vi "GetDataTypeDescription.vi"(8 "error in (no error)":errorcluster, 11 "Variant":variant) -> (0 "error out":errorcluster, 3 "String":string)   [LabVIEW 2014]
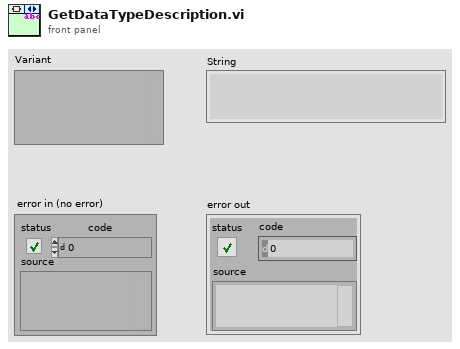
[diagram p1: front panel]
types:
  T1 = typedef "Type Descriptor__ogtk.ctl" = i16[]
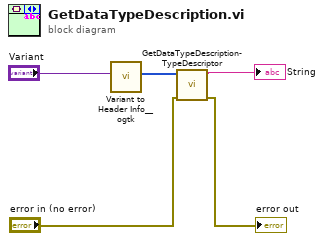
[diagram p0: block diagram]
diagram:
  n1 = call <userlib>:"Variant to Header Info__ogtk.vi"("Variant"="Variant") -> ("Type Descriptor"=w4:T1)  [unwired: 3 in, 2 out]
  n2 = call "GetDataTypeDescription-TypeDescriptor.vi"("error in (no error)"="error in (no error)", "Type Descriptor"=w4) -> ("error out"=→"error out":errorcluster, "String"=→"String":string)  [unwired: 8 in]
